vi "Output to Plotter.vi"(0 "VISA resource name":refnum<visa-resource-name>, 1 "quadrant (0 : full page)":u16(ring) items=["full page", "upper left", "lower left", "upper right", "lower right"], 3 "plot scale":bool=TRUE, 4 "plot speed":bool=TRUE, 5 "plot mkr":bool=TRUE, 6 "mkr pen number":u8=5 min=1 max=8, 7 "error in (no error)":errorcluster, 8 "plot data":bool=TRUE, 9 "plot grat":bool=TRUE, 12 "data pen number":u8=1 min=1 max=8, 13 "grat pen number":u8=3 min=1 max=8, 14 "plot mem":bool=TRUE, 15 "plot text":bool=TRUE, 16 "mem pen number":u8=2 min=1 max=8, 17 "text pen number":u8=4 min=1 max=8) -> (20 "VISA resource name out":refnum<visa-resource-name>, 27 "error out":errorcluster)   [LabVIEW 2018, in "Agilent 87XX Series.lvlib"]
doc: "This VI for the 8753B is used invoke the digital plotter on the GPIB bus.\n\n Text written with the \"write text to screen\" VI is always plotted even if everything is turned off (except the plotter of course). It is plotted in the color of the text pen."
uses:
  Agilent 87XX Series.lvlib
panel:
  # "For this VI to work properly, the address of the controlller must be \nset properly. This is done by pressing the COPY hardkey and the \nthe SET ADDRESSES softkey on the instrument front panel."
  # "ON\nOFF"
  # "FULL\nGRATICULE"
  # "ON\nOFF"
  # "FAST\nSLOW"
  # "ON\nOFF"
  # "ON\nOFF"
  # "ON\nOFF"
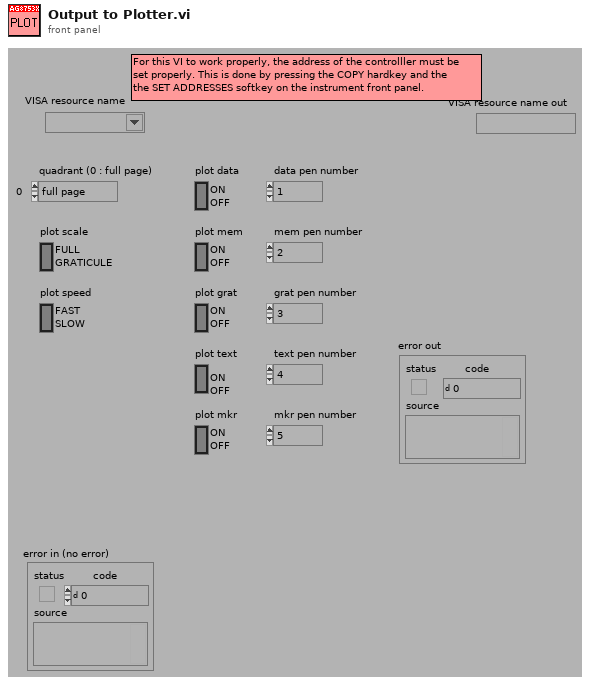
[diagram p1: front panel]
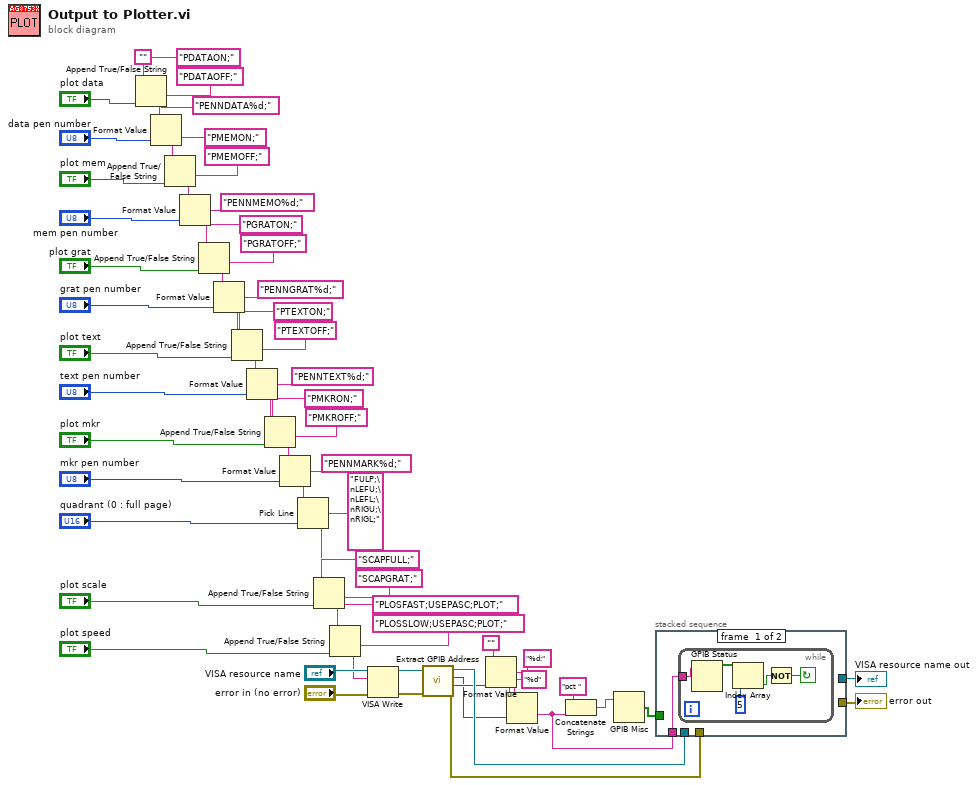
[diagram p0: block diagram]
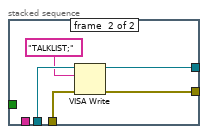
[diagram p2: hidden frame]
diagram:
  n1 = Append True/False String(1:"plot data", 2:"PDATAOFF;", 3:"PDATAON;", 4:"") -> (0:w60:string)
  n2 = Format Value(string ("")=w60, format string="PENNDATA%d;", value (0)="data pen number") -> (output string=w52:string)
  n3 = Append True/False String(1:"plot mem", 2:"PMEMOFF;", 3:"PMEMON;", 4:w52) -> (0:w55:string)
  n4 = Format Value(string ("")=w55, format string="PENNMEMO%d;", value (0)="mem pen number") -> (output string=w43:string)
  n5 = Append True/False String(1:"plot grat", 2:"PGRATOFF;", 3:"PGRATON;", 4:w43) -> (0:w49:string)
  n6 = Format Value(string ("")=w49, format string="PENNGRAT%d;", value (0)="grat pen number") -> (output string=w42:string)
  n7 = Append True/False String(1:"plot text", 2:"PTEXTOFF;", 3:"PTEXTON;", 4:w42) -> (0:w46:string)
  n8 = Format Value(string ("")=w46, format string="PENNTEXT%d;", value (0)="text pen number") -> (output string=w37:string)
  n9 = Append True/False String(1:"plot mkr", 2:"PMKROFF;", 3:"PMKRON;", 4:w37) -> (0:w39:string)
  n10 = Format Value(string ("")=w39, format string="PENNMARK%d;", value (0)="mkr pen number") -> (output string=w28:string)
  n11 = Pick Line(string ("")=w28, multi-line string="FULP;\nLEFU;\nLEFL;\nRIGU;\nRIGL;", line index="quadrant (0 : full page)") -> (output string=w23:string)
  n12 = Append True/False String(1:"plot scale", 2:"SCAPGRAT;", 3:"SCAPFULL;", 4:w23) -> (0:w20:string)
  n13 = Append True/False String(1:"plot speed", 2:"PLOSSLOW;USEPASC;PLOT;", 3:"PLOSFAST;USEPASC;PLOT;", 4:w20) -> (0:w17:string)
  n14 = VISA Write(VISA resource name="VISA resource name", write buffer=w17, error in (no error)="error in (no error)") -> (VISA resource name out=w9:refnum<visa-resource-name>, error out=w6:errorcluster)  [unwired: 1 out]
  n15 = call "Extract GPIB Address.VI"("error in (no error)"=w6, "VISA resource name"=w9) -> ("error out"=w7:errorcluster, "GPIB Board"=w2:u16, "GPIB address"=w1:u16, "VISA resource name out"=w8:refnum<visa-resource-name>)  [unwired: 6 in]
  n16 = Format Value(string ("")="", format string="%d:", value (0)=w2) -> (output string=w5:string)
  n17 = Format Value(string ("")=w5, format string="%d", value (0)=w1) -> (output string=w4:string)
  n18 = Concatenate Strings("pct ", w4) -> (w13:string)
  n19 = GPIB Misc(0:w13) -> (3:w12:bool[])  [unwired: 1 in, 2 out]
  n20 = stacked-sequence {
    tunnel: w12 -> [_ _]
    tunnel: w4 -> [w66 _]
    tunnel: w8 -> [_ w75]
    tunnel: w7 -> [_ w76]
    tunnel: [_ w73] -> w11
    tunnel: [_ w72] -> w10
    frame #0 {
      n21 = while {
        tunnel: w66 -> [w71]
        stop <- w67 continue-if-true
        n22 = GPIB Status(0:w71) -> (2:w70:bool[])  [unwired: 1 in, 3 out]
        n23 = Index Array(array=w70, index=5) -> (element=w68:bool)
        n24 = Not(x=w68) -> (.not. x?=w67:bool)
      }
    }
    frame #1 {
      n25 = VISA Write(VISA resource name=w75, write buffer="TALKLIST;", error in (no error)=w76) -> (VISA resource name out=w73:refnum<visa-resource-name>, error out=w72:errorcluster)  [unwired: 1 out]
    }
  }
  "VISA resource name out" <- w11
  "error out" <- w10
